vi "Command Line String To Path.vi"(1 "string":string) -> (0 "path":path)   [LabVIEW 2017]
doc: "Converts a <B>string</B>, describing a path in the standard command line format for the current platform, to a <B>path</B>."
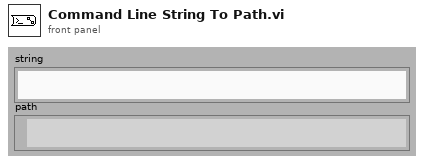
[diagram p1: front panel]
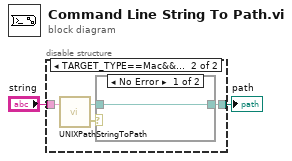
[diagram p0: block diagram]
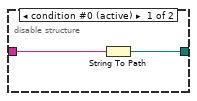
[diagram p2: hidden frame]
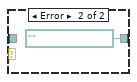
[diagram p3: hidden frame]
diagram:
  n1 = disable-structure shown="TARGET_TYPE==Mac&&TARGET_BITNESS!=64" {
    disable-tunnel: "string" -> [w4 w5]
    disable-tunnel: [w3 w8] -> w1
    frame condition #0 (active) {
      n2 = String To Path(string=w4) -> (path=w3:path)
    }
    frame condition #1 {
      n3 = call <vilib>:"UNIXPathStringToPath.vi"("UNIX Path"=w5) -> ("error out"=w7:errorcluster, "LV Path"=w6:path)  [unwired: 1 in]
      n4 = case shown="No Error" w7 {
        tunnel: w6 -> [w9 _]
        tunnel: [w9 path "" ("LV Path")] -> w8
        frame No Error {
        }
        frame Error {
        }
      }
    }
  }
  "path" <- w1
